vi "While Loop - Matching Random Number.vi"() -> ()   [LabVIEW 2016]
panel:
  out "ITERATIONS":i32
  out "OUTPUT":dbl
  in  "EMERGENCY STOP":bool
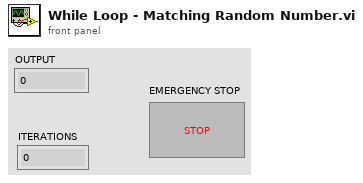
[diagram p1: front panel]
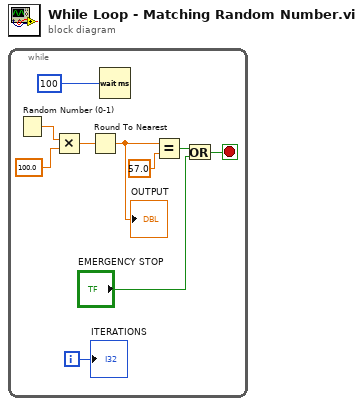
[diagram p0: block diagram]
diagram:
  n1 = while {
    i -> [w1]
    stop <- w4 stop-if-true
    n2 = Random Number (0-1)() -> (number: 0 to 1=w10:dbl)
    n3 = Multiply(x=w10, y=100.0) -> (x*y=w8:dbl)
    n4 = Round To Nearest(number=w8) -> (nearest integer value=w2:dbl)
    "OUTPUT" <- w2
    n5 = Wait (ms)(milliseconds to wait=u32 100) -> ()  [unwired: 1 out]
    n6 = Equal?(x=w2, y=57.0) -> (x = y?=w5:bool)
    n7 = Or(x=w5, y="EMERGENCY STOP") -> (x .or. y?=w4:bool)
    "ITERATIONS" <- w1
  }
